vi "Get MessageQueue.vi"(8 "error in (no error)":errorcluster, 11 "MessageQueue in":refnum<class "MessageQueue.lvclass">) -> (0 "error out":errorcluster, 2 "Native Message Queue":refnum<queue>, 3 "MessageQueue out":refnum<class "MessageQueue.lvclass">)   [LabVIEW 2017, in "LapDog.Messaging.v3.lvlib" / "MessageQueue.lvclass"]
doc: "Accessor method for the native Labview queue refnum. This method is intended for child classes to use when implementing advanced functionality.\n\nThis method ignores all input errors, passing them through unchanged."
uses:
  MessageQueue.lvclass
  Message/Message.lvclass
  MessageQueue.lvclass/MessageQueue.ctl
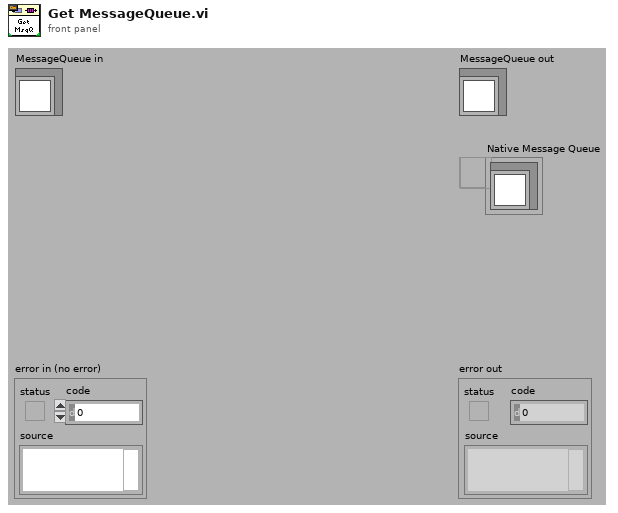
[diagram p1: front panel]
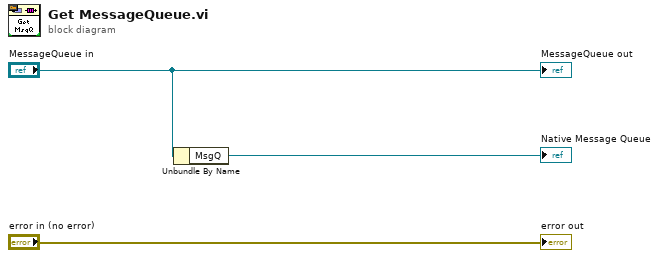
[diagram p0: block diagram]
diagram:
  n1 = Unbundle By Name("MessageQueue in") -> ("MsgQ"=→"Native Message Queue":refnum<queue>)
  "error out" <- "error in (no error)"
  "MessageQueue out" <- "MessageQueue in"
